vi "Replace Constant in VI (Array).vi"(8 "error in":errorcluster, 10 "Constant Replacement Params":T1[](array[typedef]), 11 "Original VI":path=path "C:/Users/OneEd/OneDrive/Desktop/MicroPort Job/CTDB/src/db_script/DB Select Template.vi") -> (0 "error out":errorcluster, 3 "Save as out":path=path "C:/Users/OneEd/OneDrive/Desktop/MicroPort Job/CTDB/src/db_script/DB Select Template.vi")   [LabVIEW 2021, in "EDT VI Script.lvlib"]
uses:
  EDT VI Script.lvlib
  Constant Replacement Param.ctl
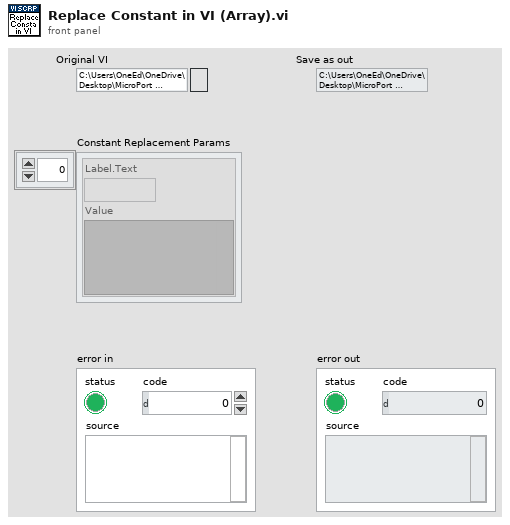
[diagram p1: front panel]
types:
  T1 = typedef "EDT VI Script.lvlib/Constant Replacement Param.ctl" = cluster{"Label.Text":string, "Value":variant}
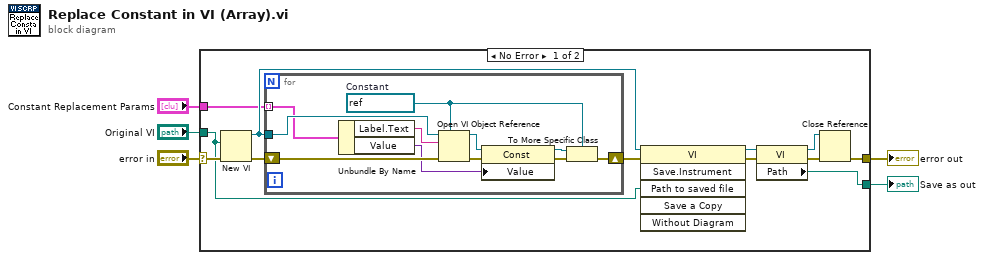
[diagram p0: block diagram]
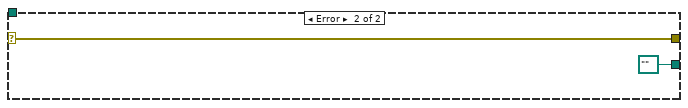
[diagram p2: hidden frame]
diagram:
  n1 = case shown="No Error" "error in" {
    selector: "error in" -> [w17 w30]
    tunnel: [w15 w30] -> w4
    tunnel: "Original VI" -> [w8 _]
    tunnel: [w11 path "" ("Path")] -> w2
    tunnel: "Constant Replacement Params" -> [w7 _]
    frame No Error {
      n2 = New VI(8:w17, 10:w8) -> (0:w16:errorcluster, 3:w14:refnum<vi>)  [unwired: 5 in]
      n3 = for {
        tunnel: w14 -> [w27]
        tunnel: w7 -> [w21] mode=indexing
        shift-right: [w22] -> w6
        shift-left: w16 -> [w28]
        w18 = refnum<vi> refnum  # Constant
        n4 = Unbundle By Name(w21) -> ("Label.Text"=w20:string, "Value"=w19:variant)
        n5 = Open VI Object Reference(7:w18, 8:w28, 10:w20, 11:w27) -> (0:w25:errorcluster, 3:w26:refnum<vi>)
        n6 = property class="Const"(reference=w26, error in=w25, "Value"=w19) -> (reference out=w24:refnum<vi>, error out=w23:errorcluster)
        n7 = To More Specific Class(target class=w18, reference=w24, error in=w23) -> (error out=w22:errorcluster)  [unwired: 1 out]
      }
      n8 = invoke class="VI" method="Save.Instrument"(reference=w14, error in=w6, "Path to saved file"=w8) -> (reference out=w10:refnum<vi>, error out=w9:errorcluster)  [unwired: 3 in, 4 out]
      n9 = property class="VI"(reference=w10, error in=w9) -> (reference out=w13:refnum<vi>, error out=w12:errorcluster, "Path"=w11:path)
      n10 = Close Reference(reference=w13, error in (no error)=w12) -> (error out=w15:errorcluster)
    }
    frame Error {
    }
  }
  "error out" <- w4
  "Save as out" <- w2
